vi "VisionGlobals.vi"() -> ()   [LabVIEW 2020]
panel:
  in  "Watchdog":dbl
  in  "YOffset":dbl
  in  "XOffset":dbl
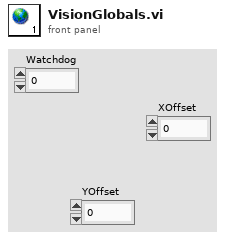
[diagram p1: front panel]
diagram:
